vi "Prog ASIC.vi"(0 "asicHandle":i32, 1 "averageOTPCurrent":dbl, 5 "progOptions":i32, 7 "sensorCurrentConsumption":dbl, 9 "minOTPCurrentRef":dbl, 11 "error in (no error)":errorcluster caption="错误输入（无错误）") -> (3 "averageOTPCurrent out":dbl, 4 "function return":i32, 8 "sensorCurrentConsumption out":dbl, 10 "minOTPCurrentRef out":dbl, 15 "error out":errorcluster caption="错误输出")   [LabVIEW 2018]
doc: "extern int __stdcall APSxProgASIC (int asicHandle, IN int progOptions, OUT double * sensorCurrentConsumption, OUT double * minOTPCurrentRef, OUT double * averageOTPCurrent);"
uses:
  APSx.dll/APSx.dll
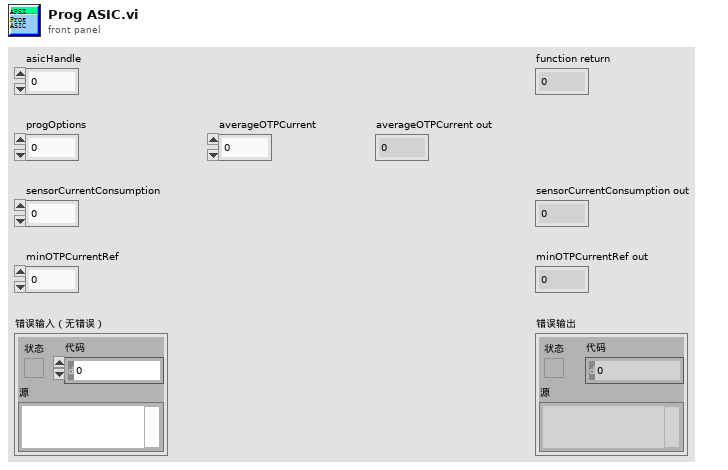
[diagram p1: front panel]
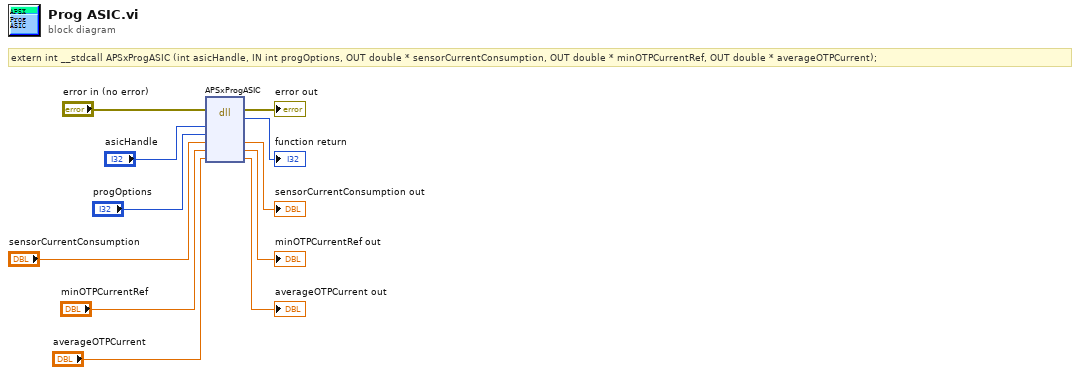
[diagram p0: block diagram]
diagram:
  # "extern int __stdcall APSxProgASIC (int asicHandle, IN int progOptions, OUT double * sensorCurrentConsumption, OUT double * minOTPCurrentRef, OUT double * averageOTPCurrent);"
  n1 = dll-call lib="PTH2[abs D项目Feng恒隆项目Labview传感器对中台SourcesAPSx.dllAPSx.*" fn="APSxProgASIC"(error in="error in (no error)", "asicHandle"="asicHandle", "progOptions"="progOptions", "sensorCurrentConsumption"="sensorCurrentConsumption", "minOTPCurrentRef"="minOTPCurrentRef", "averageOTPCurrent"="averageOTPCurrent") -> (error out=→"error out":errorcluster, →"function return":i32, "sensorCurrentConsumption"=→"sensorCurrentConsumption out":dbl, "minOTPCurrentRef"=→"minOTPCurrentRef out":dbl, "averageOTPCurrent"=→"averageOTPCurrent out":dbl)  [unwired: 4 in, 1 out]
